vi "Callback Change Direction.vi"(6 "Variant":variant, 8 "error in (no error)":errorcluster, 9 "Old Values":string[][](array[string]), 10 "object ref in":T2, 11 "Table Change":T3) -> (0 "error out":errorcluster)   [LabVIEW 2015, in "Sequencer Module editor node.lvclass"]
doc: "This VI gets called automatically when changes are made to the 'Channel Direction' column of the table and must handle changes appropriately. Register this callback using the appropriate 'Define Column' VI from the Table API."
uses:
  Sequencer Module editor node.lvclass
  <vilib>/NI/DCAF/Tag Editor Core/Table API/Table Manager/Cell Change.ctl
  <vilib>/NI/DCAF/Tag Editor Core/Table API/Table Manager/object ref.ctl
  <vilib>/NI/DCAF/Tag Editor Core/Configuration Editor/Classes/Engine Parent/Engine Parent Editor Node.lvclass
  <vilib>/NI/DCAF/Tag Editor Core/Configuration Editor/Classes/Module editor node/module editor node.lvclass
  Permissions Enum.ctl
  module/configuration/Sequencer Module configuration.lvclass
  <vilib>/NI/DCAF/Tag Editor Core/Table API/Table Manager.lvlib
  <vilib>/NI/Tag Bus Module Framework/channel/TBM channel.lvclass
  <vilib>/NI/Configuration Framework/serializable configuration/NISE_CEF_serializable configuration.lvclass
  <vilib>/NI/Module Execution Interface/Engine Configuration/engine configuration.lvclass
  <vilib>/NI/DCAF/Tag Editor Core/Table API/Table Manager/Table Manager.lvclass
panel:
  in  "Permissions":T1
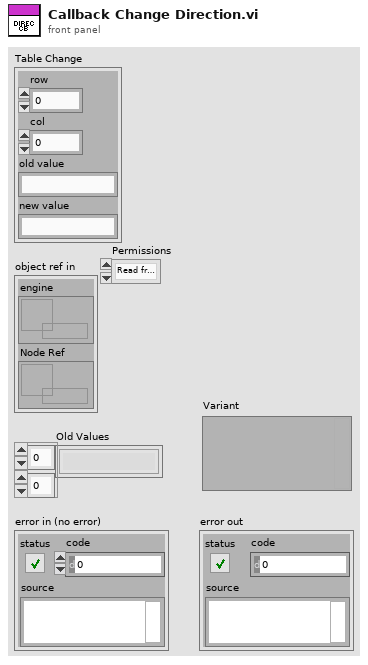
[diagram p1: front panel]
types:
  T1 = typedef "Sequencer Module editor node.lvclass/Permissions Enum.ctl" = enum16{"Read from HW", "Write to HW"}
  T2 = typedef "Table Manager.lvclass/object ref.ctl" = cluster{"engine":refnum<data-value>, "Node Ref":refnum<data-value>}
  T3 = typedef "Table Manager.lvlib/Cell Change.ctl" = cluster{"row":i32, "col":i32, "old value":string, "new value":string}
  T4 = typedef "TBM channel.lvclass/channel classification.ctl" = enum16{"input data", "output data", "processing parameter", "processing result"}
  T5 = typedef "Sequencer Module configuration.lvclass/Line.ctl" = cluster{"Sequence":refnum<class "Sequence Config.lvclass">}
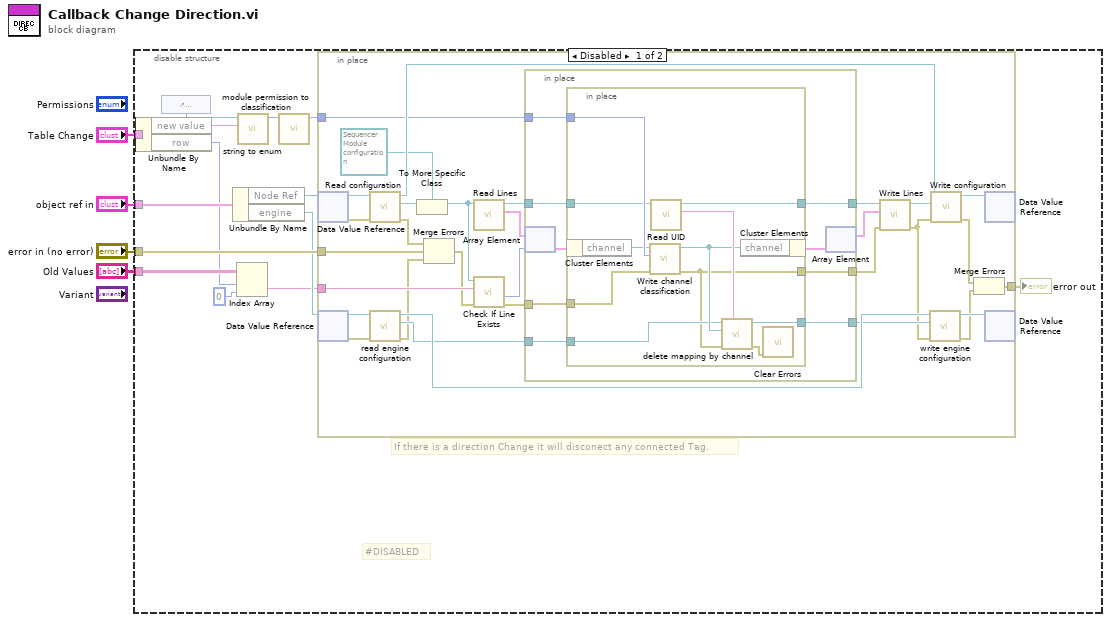
[diagram p0: block diagram]
diagram:
  n1 = disable-structure shown="Disabled" {
    disable-tunnel: "error in (no error)" -> [w17 _]
    disable-tunnel: "object ref in" -> [w16 _]
    disable-tunnel: "Table Change" -> [w13 _]
    disable-tunnel: "Old Values" -> [w8 _]
    frame Disabled {
      # "#DISABLED"
      # "If there is a direction Change it will disconect any connected Tag."
      n2 = Unbundle By Name(w13) -> ("new value"=w5:string, "row"=w6:i32)
      n3 = control-ref of="Permissions"() -> (w12:refnum<vi>)
      n4 = Unbundle By Name(w16) -> ("Node Ref"=w15:refnum<data-value>, "engine"=w14:refnum<data-value>)
      n5 = Index Array(array=w8, index (row)=w6, index (col)=0 ("disabled index (col)")) -> (element=w7:string)
      n6 = call <vilib>:"string to enum.vi"("String"=w5, "Enum"=w12) -> ("Value"=w11:i32)  [unwired: 8 in, 1 out]
      n7 = call "module permission to classification.vi"("display permissions"=w11) -> ("channel classification"=w10:T4)  [unwired: 10 in]
      n8 = in-place {
        in-place-border: [w42] -> w18
        in-place-border: w17 -> [w20]
        in-place-border: w10 -> [w30]
        in-place-border: w7 -> [w29]
        n9 = in-place-dvr #1(w15) -> (w39:refnum<class "module editor node.lvclass">, w41:errorcluster)
        n10 = in-place-dvr #2(w14) -> (w48:refnum<class "Engine Parent Editor Node.lvclass">, w49:errorcluster)
        n11 = call-dynamic "Read configuration.vi"("error in"=w41, "NISE_CEF_serializable node in"=w39) -> ("error out"=w40:errorcluster, "configuration"=w37:refnum<class "NISE_CEF_serializable configuration.lvclass">, "NISE_CEF_serializable node out"=w38:refnum<class "module editor node.lvclass">)  [unwired: 7 in]
        n12 = call <vilib>:"read engine configuration.vi"("error in"=w49, "Engine Parent Editor Node in"=w48) -> ("error out"=w19:errorcluster, "engine configuration"=w26:refnum<class "engine configuration.lvclass">, "Engine Parent Editor Node out"=w45:refnum<class "Engine Parent Editor Node.lvclass">)  [unwired: 7 in]
        n13 = To More Specific Class(target class=refnum<class "Sequencer Module configuration.lvclass"> refnum ("tag bus configurable plugin module configuration"), reference=w37) -> (specific class reference=w34:refnum<class "Sequencer Module configuration.lvclass">)  [unwired: 1 in, 1 out]
        n14 = Merge Errors(w40, w20, w19) -> (w24:errorcluster)
        n15 = call "Read Lines.vi"("Sequencer Module configuration in"=w34) -> ("Lines"=w33:T5[], "Sequencer Module configuration out"=w28:refnum<class "Sequencer Module configuration.lvclass">)  [unwired: 8 in, 1 out]
        n16 = call-dynamic "Check If Line Exists.vi"("error in"=w24, "Name to Locate"=w29, "Sequencer Module configuration in"=w34) -> ("error out"=w23:errorcluster, "Index"=w31:i32)  [unwired: 4 in, 3 out]
        n17 = in-place {
          in-place-border: w30 -> [w56]
          in-place-border: w28 -> [w55]
          in-place-border: [w54] -> w27
          in-place-border: w26 -> [w53]
          in-place-border: [w52] -> w25
          in-place-border: w23 -> [w51]
          in-place-border: [w50] -> w22
          n18 = in-place-array #3(w33, w31) -> (w58:T5)
          n19 = in-place {
            in-place-border: w56 -> [w69]
            in-place-border: w55 -> [w68]
            in-place-border: [w67] -> w54
            in-place-border: w53 -> [w61]
            in-place-border: [w65] -> w52
            in-place-border: w51 -> [w62]
            in-place-border: [w59] -> w50
            n20 = in-place-cluster #4(w58) -> ("channel"=w66:refnum<class "TBM channel.lvclass">)
            n21 = call <vilib>:"Write channel classification.vi"("error in"=w62, "channel classification"=w69, "channel in"=w66) -> ("error out"=w59:errorcluster, "channel out"=w63:refnum<class "TBM channel.lvclass">)  [unwired: 7 in]
            n22 = call <vilib>:"Read UID.vi"("configuration in"=w68) -> ("instance id"=w64:string, "configuration out"=w67:refnum<class "Sequencer Module configuration.lvclass">)  [unwired: 8 in, 1 out]
            n23 = call <vilib>:"delete mapping by channel.vi"("owner ID"=w64, "error in"=w59, "channel"=w63, "engine configuration in"=w61) -> ("error out"=w60:errorcluster, "engine configuration out"=w65:refnum<class "engine configuration.lvclass">)  [unwired: 6 in]
            n24 = in-place-cluster #4("channel"=w63) -> (w57:T5)
            n25 = call <vilib>:"Clear Errors.vi"("error in (no error)"=w60) -> ()  [unwired: 5 in, 2 out]
          }
          n26 = in-place-array #3(w57) -> (w32:T5[])  [unwired: 1 out]
        }
        n27 = call "Write Lines.vi"("error in (no error)"=w22, "Lines"=w32, "Sequencer Module configuration in"=w27) -> ("error out"=w21:errorcluster, "Sequencer Module configuration out"=w35:refnum<class "Sequencer Module configuration.lvclass">)  [unwired: 7 in]
        n28 = call <vilib>:"write engine configuration.vi"("error in"=w21, "engine configuration"=w25, "Engine Parent Editor Node in"=w45) -> ("error out"=w44:errorcluster, "Engine Parent Editor Node out"=w47:refnum<class "Engine Parent Editor Node.lvclass">)  [unwired: 7 in]
        n29 = call-dynamic "Write configuration.vi"("error in"=w21, "configuration"=w35, "NISE_CEF_serializable node in"=w38) -> ("error out"=w43:errorcluster, "NISE_CEF_serializable node out"=w46:refnum<class "module editor node.lvclass">)  [unwired: 7 in]
        n30 = Merge Errors(w43, w44) -> (w42:errorcluster)
        n31 = in-place-dvr #1(w46) -> ()  [unwired: 2 out]
        n32 = in-place-dvr #2(w47) -> ()  [unwired: 2 out]
      }
      "error out" <- w18
    }
    frame Enabled {
    }
  }
